vi "Sort Incoming Parameter.vi"(8 "Error In":errorcluster, 10 "Aircraft ID":u8, 11 "Param Value":T1) -> (0 "Error Out":errorcluster)   [LabVIEW 2014]
uses:
  Controls/MAVLink Recieved Param.ctl
  Aircraft Information/Sub VI/Set Aircraft RC.vi
  Aircraft Information/Sub VI/Get Aircraft RC.vi
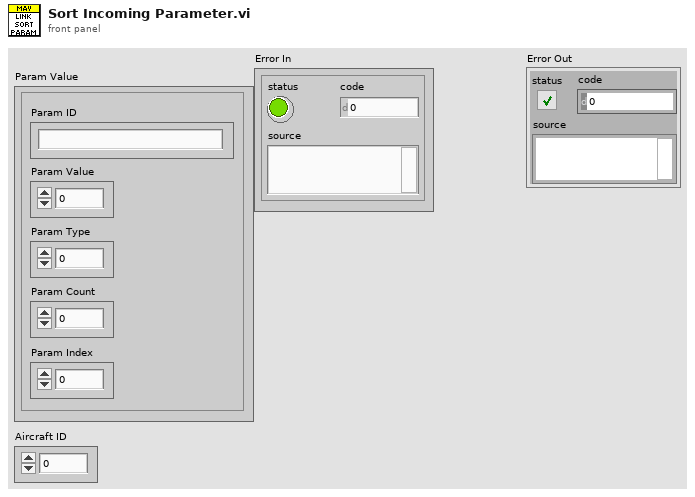
[diagram p1: front panel]
types:
  T1 = typedef "MAVLink Recieved Param.ctl" = cluster{"Param ID":string, "Param Value":sgl, "Param Type":u8, "Param Count":u16, "Param Index":u16}
  T2 = typedef "Aircraft RC Data.ctl" = cluster{"Channel 1 Min":i16, "Channel 1 Max":i16, "Channel 2 Min":i16, "Channel 2 Max":i16, "Channel 3 Min":i16, "Channel 3 Max":i16, "Channel 4 Min":i16, "Channel 4 Max":i16}
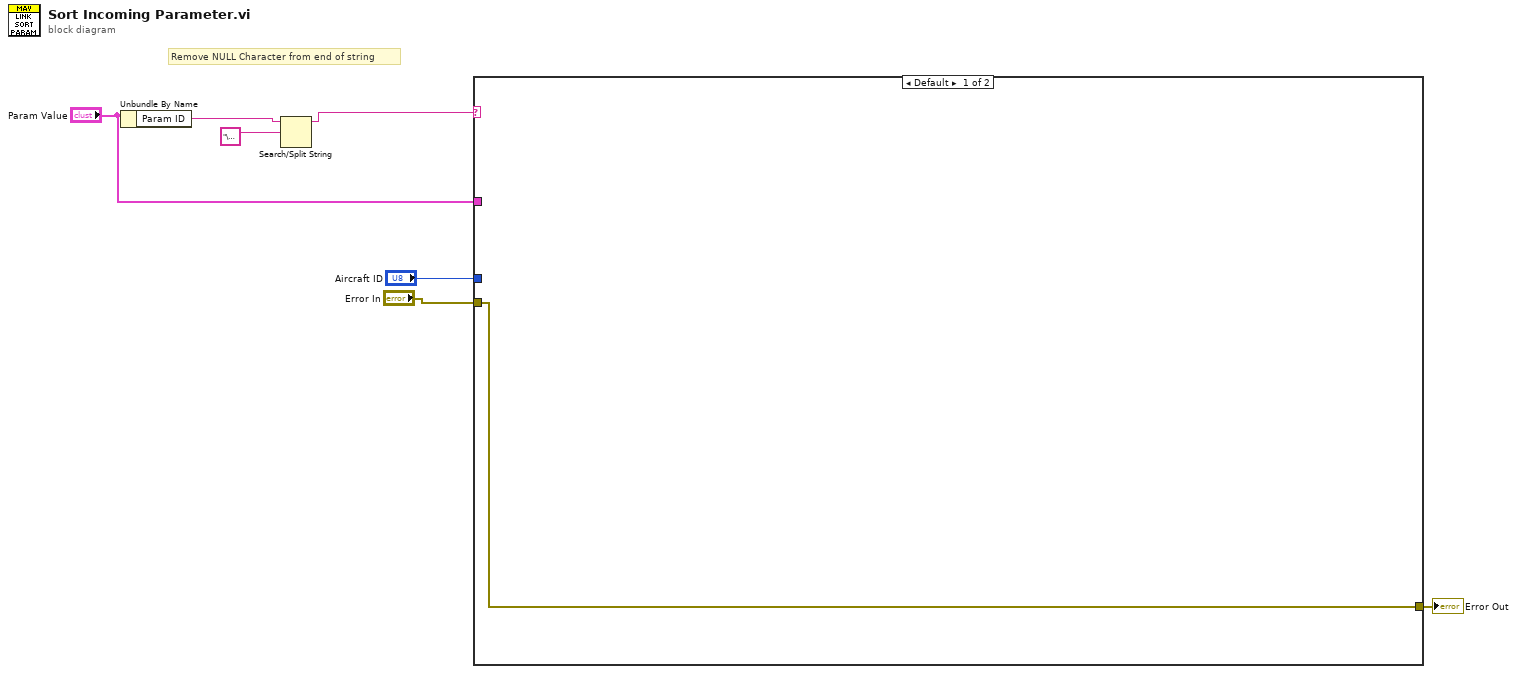
[diagram p0: block diagram]
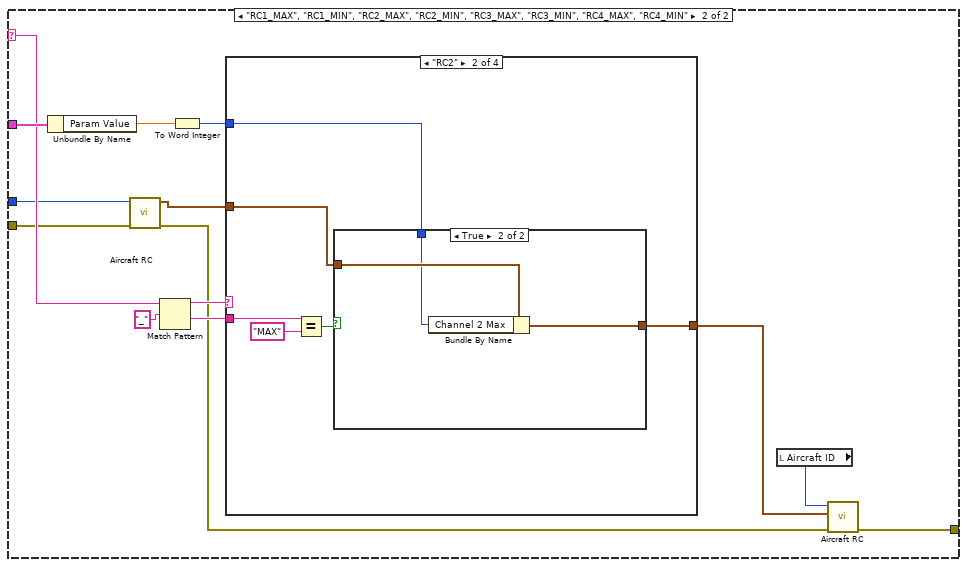
[diagram p2: hidden frame]
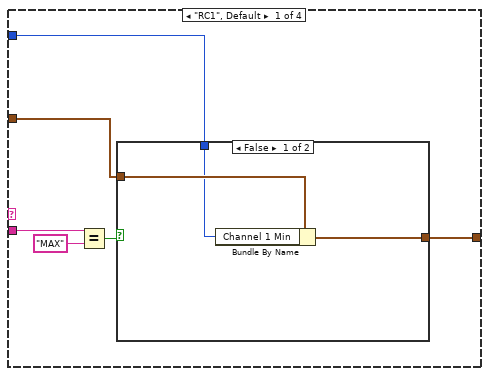
[diagram p3: hidden frame]
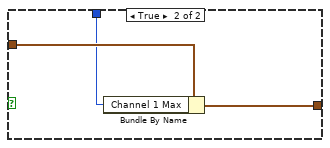
[diagram p4: hidden frame]
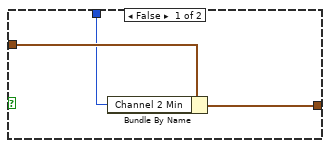
[diagram p5: hidden frame]
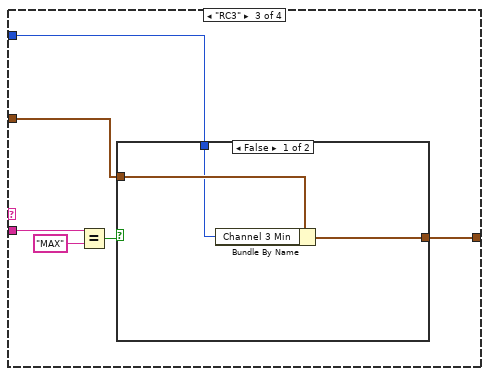
[diagram p6: hidden frame]
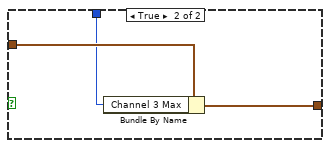
[diagram p7: hidden frame]
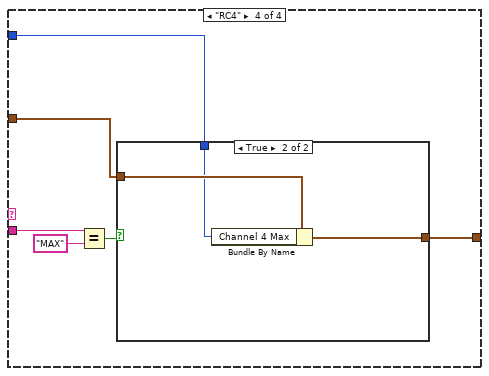
[diagram p8: hidden frame]
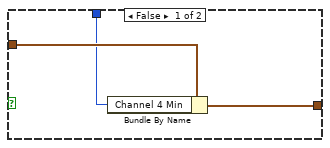
[diagram p9: hidden frame]
diagram:
  # "Remove NULL Character from end of string"
  n1 = Unbundle By Name("Param Value") -> ("Param ID"=w6:string)
  n2 = Search/Split String(string=w6, search string/char (-)="\u0000") -> (substring before match=w5:string)  [unwired: 1 in, 2 out]
  n3 = case shown="Default" w5 {
    selector: w5 -> [_ w16]
    tunnel: "Param Value" -> [_ w22]
    tunnel: "Aircraft ID" -> [_ w14]
    tunnel: "Error In" -> [w8 w11]
    tunnel: [w8 w9] -> w1
    frame Default {
    }
    frame "RC1_MAX", "RC1_MIN", "RC2_MAX", "RC2_MIN", "RC3_MAX", "RC3_MIN", "RC4_MAX", "RC4_MIN" {
      n4 = Unbundle By Name(w22) -> ("Param Value"=w18:sgl)
      n5 = call-poly "Aircraft RC.vi"("Error In"=w11, "Aircraft ID"=w14) -> ("Error Out"=w10:errorcluster, "Aircraft RC Data"=w15:T2)  [unwired: 8 in]
      n6 = Match Pattern(string=w16, regular expression="_") -> (before substring=w20:string, after substring=w19:string)  [unwired: 1 in, 2 out]
      n7 = To Word Integer(number=w18) -> (16bit integer=w17:i16)
      n8 = case shown="\"RC2\"" w20 {
        tunnel: w19 -> [w28 w40 w52 w64]
        tunnel: w15 -> [w25 w37 w49 w61]
        tunnel: w17 -> [w24 w36 w48 w60]
        tunnel: [w23 w35 w47 w59] -> w13
        frame "RC1", Default {
          n9 = Equal?(x=w28, y="MAX") -> (x = y?=w26:bool)
          n10 = case shown="False" w26 {
            tunnel: w25 -> [w31 w34]
            tunnel: w24 -> [w30 w32]
            tunnel: [w29 w33] -> w23
            frame False {
              n11 = Bundle By Name(cluster=w31, "Channel 1 Min"=w30) -> (w29:T2)
            }
            frame True {
              n12 = Bundle By Name(cluster=w34, "Channel 1 Max"=w32) -> (w33:T2)
            }
          }
        }
        frame "RC2" {
          n13 = Equal?(x=w40, y="MAX") -> (x = y?=w38:bool)
          n14 = case shown="True" w38 {
            tunnel: w37 -> [w43 w46]
            tunnel: w36 -> [w42 w44]
            tunnel: [w41 w45] -> w35
            frame False {
              n15 = Bundle By Name(cluster=w43, "Channel 2 Min"=w42) -> (w41:T2)
            }
            frame True {
              n16 = Bundle By Name(cluster=w46, "Channel 2 Max"=w44) -> (w45:T2)
            }
          }
        }
        frame "RC3" {
          n17 = Equal?(x=w52, y="MAX") -> (x = y?=w50:bool)
          n18 = case shown="False" w50 {
            tunnel: w49 -> [w55 w58]
            tunnel: w48 -> [w54 w56]
            tunnel: [w53 w57] -> w47
            frame False {
              n19 = Bundle By Name(cluster=w55, "Channel 3 Min"=w54) -> (w53:T2)
            }
            frame True {
              n20 = Bundle By Name(cluster=w58, "Channel 3 Max"=w56) -> (w57:T2)
            }
          }
        }
        frame "RC4" {
          n21 = Equal?(x=w64, y="MAX") -> (x = y?=w62:bool)
          n22 = case shown="True" w62 {
            tunnel: w61 -> [w67 w70]
            tunnel: w60 -> [w66 w68]
            tunnel: [w65 w69] -> w59
            frame False {
              n23 = Bundle By Name(cluster=w67, "Channel 4 Min"=w66) -> (w65:T2)
            }
            frame True {
              n24 = Bundle By Name(cluster=w70, "Channel 4 Max"=w68) -> (w69:T2)
            }
          }
        }
      }
      n25 = local read "Aircraft ID"() -> (w12:u8)
      n26 = call-poly "Aircraft RC.vi"("Error In"=w10, "Aircraft RC Data"=w13, "Aircraft ID"=w12) -> ("Error Out"=w9:errorcluster)  [unwired: 8 in]
    }
  }
  "Error Out" <- w1
